vi "hitter1.vi"(1 "increments":dbl, 2 "+ or -":dbl, 3 "NXT/EV3":T1) -> (0 "NXT/EV3 2":T1)   [LabVIEW 2016]
uses:
  <vilib>/NXT/Subs/LVHSConnector.ctl
  <vilib>/NXT/LegoClasses/BrickReference/BrickReference.lvclass
  <vilib>/NXT/Block Support/NXT_InputPort.ctl
  <vilib>/NXT/Block Support/NXT_OutputPort.ctl
  <vilib>/NXT/NXTIO Xnodes/NXTIONodeSubVIs/NXTMotorRunDistance.vi
  <vilib>/NXT/NXTIO Xnodes/NXTIONodeSubVIs/NXTMoveMotors.vi
  <vilib>/NXT/Dual Mode Library/Waits/Wait_Touch.vi
  <vilib>/NXT/NXTIO Xnodes/NXTIONodeSubVIs/NXTStopMotors.vi
  <vilib>/NXT/NXTIO Xnodes/AddressXNode/NXTIOAddress.xnode
  <vilib>/NXT/NXTIO Xnodes/NXTIOXNode/NXTIO.xnode
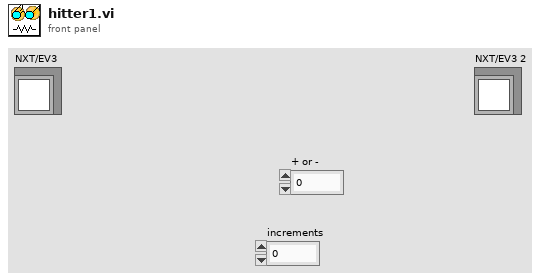
[diagram p1: front panel]
types:
  T1 = typedef "LVHSConnector.ctl" = refnum<class "BrickReference.lvclass">
  T2 = typedef "NXT_InputPort.ctl" = u32
  T3 = typedef "NXT_OutputPort.ctl" = u8
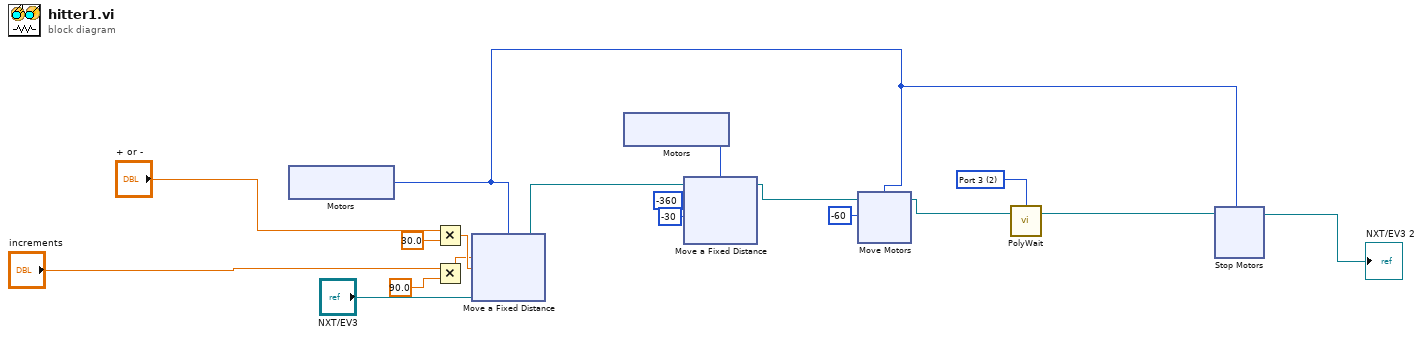
[diagram p0: block diagram]
diagram:
  w1 = T2 2 items=["Port 1", "Port 2", "Port 3", "Port 4"] ("Port (Port 1)")
  n1 = xnode "Motors"() -> ("Motor"=w5:T3)
  n2 = Multiply(x="+ or -", y=30.0) -> (x*y=w12:dbl)
  n3 = Multiply(x="increments", y=90.0) -> (x*y=w8:dbl)
  n4 = xnode "Move a Fixed Distance"("Speed 1"=w12, "Distance 1"=w8, "Motors"=w5, "NXT/EV3"="NXT/EV3") -> ("NXT/EV3"=w18:T1)
  n5 = xnode "Motors"() -> ("Motor"=w17:T3)
  n6 = xnode "Move a Fixed Distance"("Speed 1"=i8 -30, "Distance 1"=-360, "Motors"=w17, "NXT/EV3"=w18) -> ("NXT/EV3"=w7:T1)
  n7 = xnode "Move Motors"("Power/Speed 1"=i8 -60, "Motors"=w5, "NXT/EV3"=w7) -> ("NXT/EV3"=w3:T1)
  n8 = call-poly <vilib>:"PolyWait.vi"("NXT/EV3"=w3, "Port (Port 1)"=w1) -> ("NXT/EV3"=w2:T1)  [unwired: 2 in]
  n9 = xnode "Stop Motors"("Motors"=w5, "NXT/EV3"=w2) -> ("NXT/EV3"=→"NXT/EV3 2":T1)
